vi "host.vi"() -> ()   [LabVIEW 2020]
uses:
  <vilib>/FPGAPlugInAG/cRIO-9035/niLvFpga_Open_cRIO-9035.vi
  <vilib>/rvi/interface/common/dynamic/niFpgaDynamicAddResources.vi
  <vilib>/rvi/interface/common/niFpgaWaitOnOcc.vi
  <vilib>/Utility/error.llb/Error Cluster From Error Code.vi
  <vilib>/rvi/errors/niLvFpgaAdjustHostInterfaceError.vi
  <vilib>/FPGAPlugInAG/Dynamic/niLvFpga_Run_Dynamic.vi
  <vilib>/FPGAPlugInAG/Dynamic/niLvFpga_Close_Dynamic.vi
  <vilib>/rvi/interface/nirviOpenFPGA/nirviOpenFPGA.xnode
  FPGA Bitfiles/fftfpgaapplicati_FPGATarget_FFT2_yc4HosK7ewc.lvbitx
  FFT.vi
  <vilib>/rvi/interface/nirviMethod/nirviMethod.xnode
  <vilib>/rvi/interface/nirviCloseFPGA/nirviCloseFPGA.xnode
  <vilib>/rvi/errors/niLvFpgaMergeErrorWithErrorCode.vi
  <vilib>/FPGAPlugInAG/Dynamic/niLvFpga_ReadFifo_Dynamic.vi
  <vilib>/Analysis/NI_AALPro.lvlib
  <vilib>/FPGAPlugInAG/Dynamic/niLvFpga_StartFifo_Dynamic.vi
  <vilib>/FPGAPlugInAG/Dynamic/niLvFpga_ConfigureFifo_Dynamic.vi
  <vilib>/FPGAPlugInAG/Dynamic/niLvFpga_WriteFifo_Dynamic.vi
panel:
  out "target to hostActual Depth 4":u32
  out "imag_Actual Depth 3":u32
  out "real actual depth":u32
  out "Actual Depth host to target":u32
  out "imaginary":fxp<+/-,32,21>[](array[numeric])
  out "real remain 1st":u32
  out "img remain 1st":u32
  out "data collrection remain 2nd":u32
  out "data collection remain 1st":u32
  out "FF T time remain 2nd":u32
  out "FFt time remain 1st":u32
  out "real remain 2nd":u32
  out "img remain 2nd":u32
  out "target to host remain 2nd":u32
  out "Empty Elements Remaining\nhost to target":u32
  out "signal_target_to_host_fixed size(s)":i32
  out "target to host remain 1st":u32
  out "Array":fxp<+/-,24,7>[](array[numeric])
  out "signal target to host":dbl[][](graph)
  out "data collection time":u32[](array[numeric])
  out "FFT time":u32[](array[numeric])
  out "signal_target_to_host_fixed":fxp<+/-,24,7>[](array[numeric])
  out "real array size":i32
  out "real Fixed":fxp<+/-,32,21>[](array[numeric])
  out "detrend acc":dbl[](graph)
  out "acc":dbl[](graph)
  out "samples":i32
  out "Waveform Graph":dbl[][](graph)
  out "input signal":T1(graph)
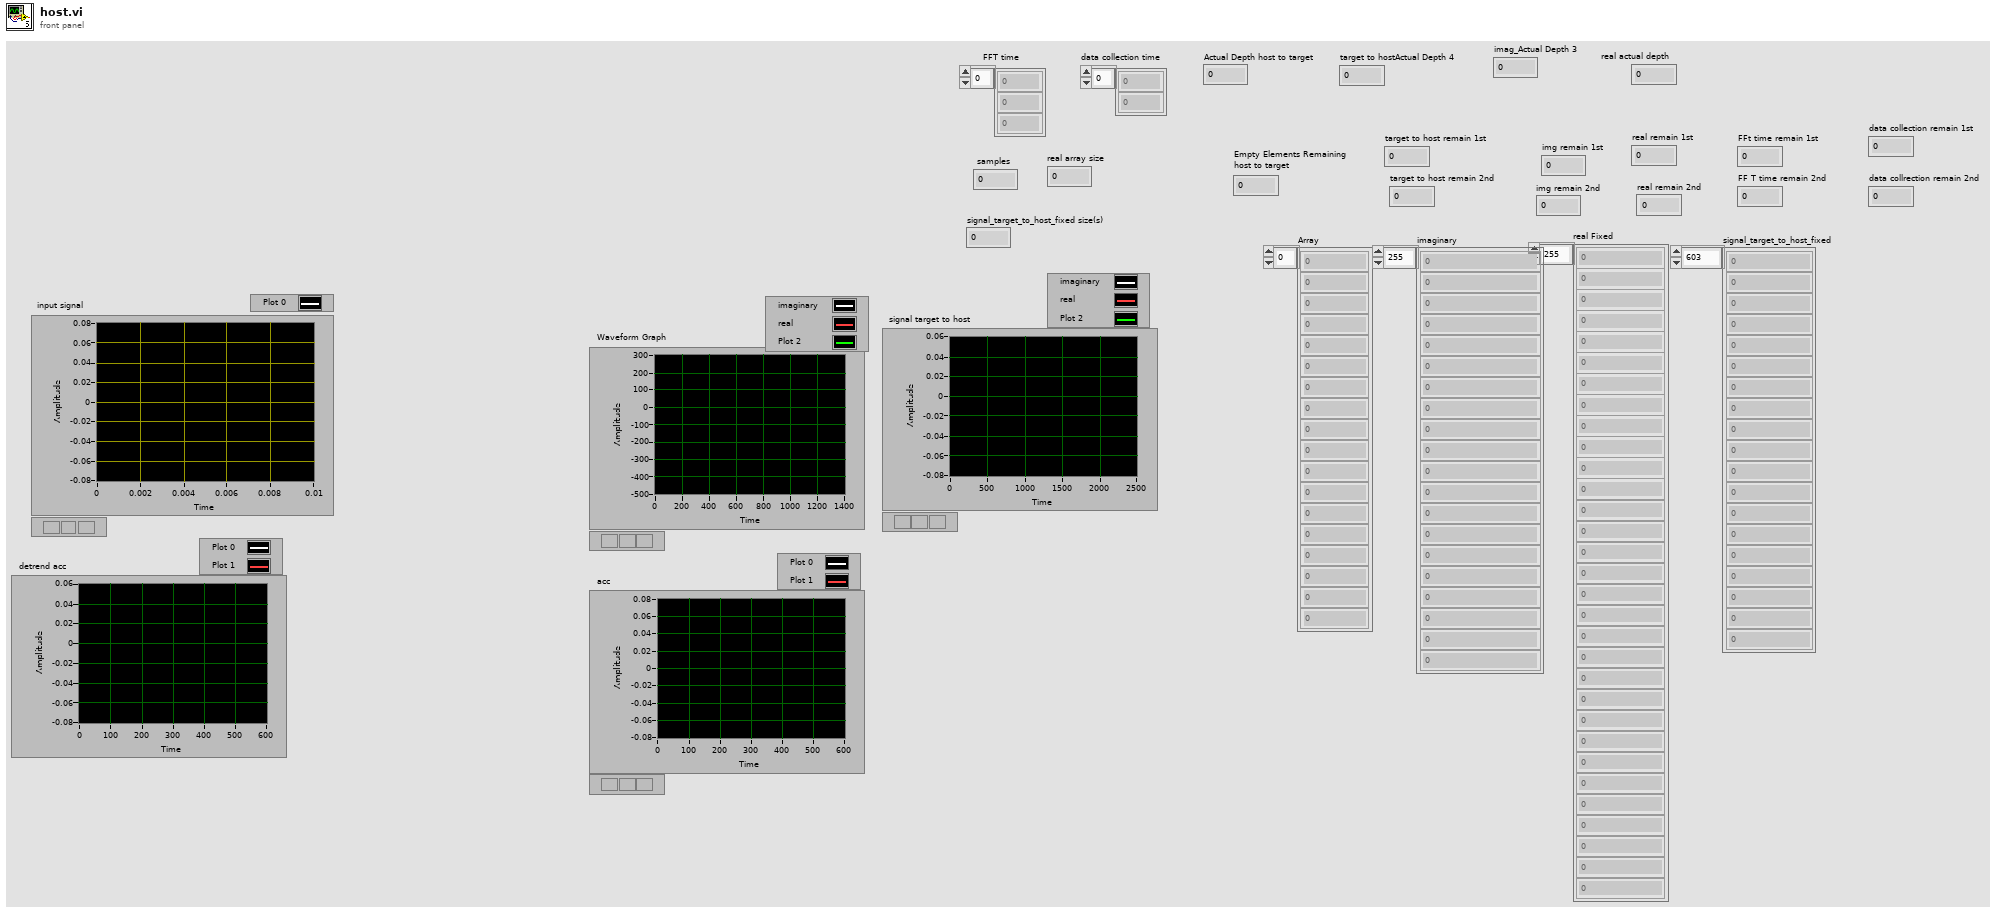
[diagram p1: front panel]
types:
  T1 = cluster{"array type (2D Dbl)":dbl[], "array type (2D Dbl)":dbl[]}
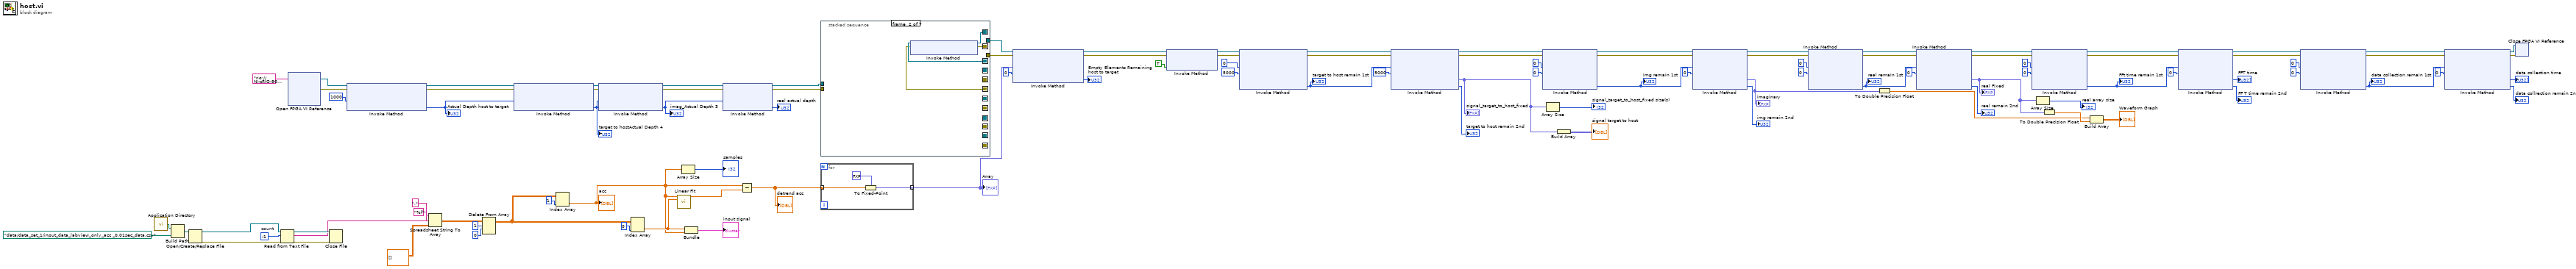
[diagram p0: block diagram]
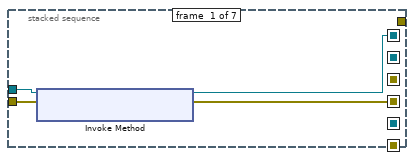
[diagram p2: hidden frame]
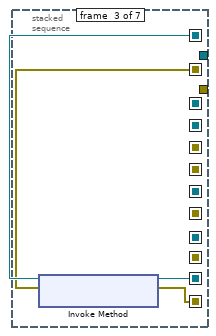
[diagram p3: hidden frame]
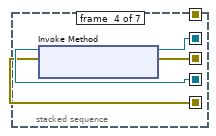
[diagram p4: hidden frame]
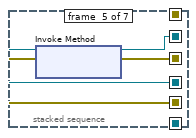
[diagram p5: hidden frame]
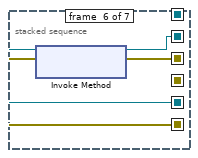
[diagram p6: hidden frame]
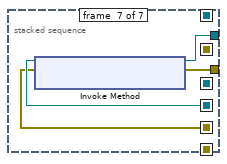
[diagram p7: hidden frame]
diagram:
  w97 = -1  # count
  n1 = call <vilib>:"Application Directory.vi"() -> ("Application Directory"=w101:path)
  n2 = Build Path(base path=w101, name or relative path=path "data/data_set_1/input_data_labview_only_acc _0.01sec_data.csv" ("default name")) -> (appended path=w100:path)
  n3 = Open/Create/Replace File(file path (use dialog)=w100) -> (refnum out=w105:refnum<file>, error out=w106:errorcluster)  [unwired: 5 in, 1 out]
  n4 = Read from Text File(file (use dialog)=w105, count=w97, error in=w106) -> (refnum out=w104:refnum<file>, text=w102:string, error out=w103:errorcluster)  [unwired: 1 in, 1 out]
  n5 = xnode "Open FPGA VI Reference"("resource name"=tag "rio://NI-cRIO-9035-01B68DD0/RIO0") -> ("FPGA VI Reference Out"=w10:refnum<k20>, "error out"=w9:errorcluster)  [unwired: 1 in]
  n6 = Close File(refnum=w104, error in=w103) -> ()  [unwired: 2 out]
  n7 = xnode "Invoke Method"("FPGA VI Reference In"=w10, "error in"=w9, "Requested Depth"=u32 1000) -> ("FPGA VI Reference Out"=w8:refnum<k20>, "error out"=w7:errorcluster, "Actual Depth"=w14:u32)
  "Actual Depth host to target" <- w14
  n8 = Spreadsheet String To Array(delimiter (Tab)=",", format string="%f", spreadsheet string=w102, array type (2D Dbl)=dbl[][] []) -> (array=w94:dbl[][])
  n9 = Delete From Array(array=w94, length=1, index (row)=0) -> (array with subset deleted=w89:dbl[][])  [unwired: 1 in, 1 out]
  n10 = xnode "Invoke Method"("FPGA VI Reference In"=w8, "error in"=w7, "Requested Depth"=w14) -> ("FPGA VI Reference Out"=w6:refnum<k20>, "error out"=w5:errorcluster, "Actual Depth"=w13:u32)
  "target to hostActual Depth 4" <- w13
  n11 = Index Array(array=w89, index (col)=1 ("disabled index (col)")) -> (element=w71:dbl[])  [unwired: 1 in]
  "acc" <- w71
  n12 = xnode "Invoke Method"("FPGA VI Reference In"=w6, "error in"=w5, "Requested Depth"=w13) -> ("FPGA VI Reference Out"=w4:refnum<k20>, "error out"=w3:errorcluster, "Actual Depth"=w12:u32)
  "imag_Actual Depth 3" <- w12
  n13 = Index Array(array=w89, index (col)=0 ("disabled index (col)")) -> (element=w74:dbl[])  [unwired: 1 in]
  n14 = call <vilib>:"Linear Fit.vi"("Y"=w71, "X"=w74) -> ("Best Linear Fit"=w72:dbl[])  [unwired: 9 in, 4 out]
  n15 = Array Size(array=w71) -> (size(s)=→"samples":i32)
  n16 = Bundle("array type (2D Dbl)"=w74, "array type (2D Dbl)"=w71) -> (→"input signal":T1)  [unwired: 1 in]
  n17 = xnode "Invoke Method"("FPGA VI Reference In"=w4, "error in"=w3, "Requested Depth"=w12) -> ("FPGA VI Reference Out"=w2:refnum<k20>, "error out"=w1:errorcluster, "Actual Depth"=→"real actual depth":u32)
  n18 = Subtract(x=w71, y=w72) -> (x-y=w73:dbl[])
  "detrend acc" <- w73
  n19 = stacked-sequence {
    seq-local: [w108 _ _ _ _ _ _] -> [_ w114 _ _ _ _ _]
    seq-local: [w107 _ _ _ _ _ _] -> [_ w113 _ _ _ _ _]
    seq-local: [_ w112 _ _ _ _ _] -> [_ _ w118 _ _ _ _]
    seq-local: [_ w111 _ _ _ _ _] -> [_ _ w117 _ _ _ _]
    seq-local: [_ _ w116 _ _ _ _] -> [_ _ _ w122 _ _ _]
    seq-local: [_ _ w115 _ _ _ _] -> [_ _ _ w121 _ _ _]
    seq-local: [_ _ _ w120 _ _ _] -> [_ _ _ _ w126 _ _]
    seq-local: [_ _ _ w119 _ _ _] -> [_ _ _ _ w125 _ _]
    seq-local: [_ _ _ _ w124 _ _] -> [_ _ _ _ _ w130 _]
    seq-local: [_ _ _ _ w123 _ _] -> [_ _ _ _ _ w129 _]
    seq-local: [_ _ _ _ _ w128 _] -> [_ _ _ _ _ _ w134]
    seq-local: [_ _ _ _ _ w127 _] -> [_ _ _ _ _ _ w133]
    tunnel: w2 -> [w110 _ _ _ _ _ _]
    tunnel: w1 -> [w109 _ _ _ _ _ _]
    tunnel: [_ _ _ _ _ _ w132] -> w34
    tunnel: [_ _ _ _ _ _ w131] -> w33
    frame #0 {
      n20 = xnode "Invoke Method"("FPGA VI Reference In"=w110, "error in"=w109) -> ("FPGA VI Reference Out"=w108:refnum<k20>, "error out"=w107:errorcluster)
    }
    frame #1 {
      n21 = xnode "Invoke Method"("FPGA VI Reference In"=w114, "error in"=w113) -> ("FPGA VI Reference Out"=w112:refnum<k20>, "error out"=w111:errorcluster)
    }
    frame #2 {
      n22 = xnode "Invoke Method"("FPGA VI Reference In"=w118, "error in"=w117) -> ("FPGA VI Reference Out"=w116:refnum<k20>, "error out"=w115:errorcluster)
    }
    frame #3 {
      n23 = xnode "Invoke Method"("FPGA VI Reference In"=w122, "error in"=w121) -> ("FPGA VI Reference Out"=w120:refnum<k20>, "error out"=w119:errorcluster)
    }
    frame #4 {
      n24 = xnode "Invoke Method"("FPGA VI Reference In"=w126, "error in"=w125) -> ("FPGA VI Reference Out"=w124:refnum<k20>, "error out"=w123:errorcluster)
    }
    frame #5 {
      n25 = xnode "Invoke Method"("FPGA VI Reference In"=w130, "error in"=w129) -> ("FPGA VI Reference Out"=w128:refnum<k20>, "error out"=w127:errorcluster)
    }
    frame #6 {
      n26 = xnode "Invoke Method"("FPGA VI Reference In"=w134, "error in"=w133) -> ("FPGA VI Reference Out"=w132:refnum<k20>, "error out"=w131:errorcluster)
    }
  }
  n27 = for {
    tunnel: [w136] -> w62 mode=indexing
    tunnel: w73 -> [w135] mode=indexing
    n28 = To Fixed-Point(fixed-point type=fxp<+/-,24,7> 0.0 ("f"), number=w135) -> (fixed-point=w136:fxp<+/-,24,7>)
  }
  "Array" <- w62
  n29 = xnode "Invoke Method"("FPGA VI Reference In"=w34, "error in"=w33, "Data"=w62, "Timeout (ms)"=0) -> ("FPGA VI Reference Out"=w86:refnum<k20>, "error out"=w85:errorcluster, "Empty Elements Remaining"=→"Empty Elements Remaining\nhost to target":u32)
  n30 = xnode "Invoke Method"("FPGA VI Reference In"=w86, "error in"=w85, "Wait Until Done (F)"=TRUE) -> ("FPGA VI Reference Out"=w63:refnum<k20>, "error out"=w64:errorcluster)
  n31 = xnode "Invoke Method"("FPGA VI Reference In"=w63, "error in"=w64, "Number of Elements"=u32 0, "Timeout (ms)"=5000) -> ("FPGA VI Reference Out"=w66:refnum<k20>, "error out"=w65:errorcluster, "Elements Remaining"=w31:u32)  [unwired: 1 out]
  "target to host remain 1st" <- w31
  n32 = xnode "Invoke Method"("FPGA VI Reference In"=w66, "error in"=w65, "Number of Elements"=w31, "Timeout (ms)"=5000) -> ("FPGA VI Reference Out"=w29:refnum<k20>, "error out"=w28:errorcluster, "Data"=w43:fxp<+/-,24,7>[], "Elements Remaining"=→"target to host remain 2nd":u32)
  "signal_target_to_host_fixed" <- w43
  n33 = xnode "Invoke Method"("FPGA VI Reference In"=w29, "error in"=w28, "Number of Elements"=u32 0, "Timeout (ms)"=0) -> ("FPGA VI Reference Out"=w25:refnum<k20>, "error out"=w24:errorcluster, "Elements Remaining"=w23:u32)  [unwired: 1 out]
  "img remain 1st" <- w23
  n34 = Array Size(array=w43) -> (size(s)=→"signal_target_to_host_fixed size(s)":i32)
  n35 = Build Array(w43) -> (→"signal target to host":fxp<+/-,24,7>[][])
  n36 = xnode "Invoke Method"("FPGA VI Reference In"=w25, "error in"=w24, "Number of Elements"=w23, "Timeout (ms)"=0) -> ("FPGA VI Reference Out"=w22:refnum<k20>, "error out"=w21:errorcluster, "Data"=w30:fxp<+/-,32,21>[], "Elements Remaining"=→"img remain 2nd":u32)
  "imaginary" <- w30
  n37 = xnode "Invoke Method"("FPGA VI Reference In"=w22, "error in"=w21, "Number of Elements"=u32 0, "Timeout (ms)"=0) -> ("FPGA VI Reference Out"=w20:refnum<k20>, "error out"=w19:errorcluster, "Elements Remaining"=w16:u32)  [unwired: 1 out]
  "real remain 1st" <- w16
  n38 = To Double Precision Float(number=w30) -> (double precision float=w67:dbl[])
  n39 = xnode "Invoke Method"("FPGA VI Reference In"=w20, "error in"=w19, "Number of Elements"=w16, "Timeout (ms)"=0) -> ("FPGA VI Reference Out"=w81:refnum<k20>, "error out"=w80:errorcluster, "Data"=w69:fxp<+/-,32,21>[], "Elements Remaining"=→"real remain 2nd":u32)
  "real Fixed" <- w69
  n40 = xnode "Invoke Method"("FPGA VI Reference In"=w81, "error in"=w80, "Number of Elements"=u32 0, "Timeout (ms)"=0) -> ("FPGA VI Reference Out"=w59:refnum<k20>, "error out"=w58:errorcluster, "Elements Remaining"=w57:u32)  [unwired: 1 out]
  "FFt time remain 1st" <- w57
  n41 = Array Size(array=w69) -> (size(s)=→"real array size":i32)
  n42 = To Double Precision Float(number=w69) -> (double precision float=w68:dbl[])
  n43 = Build Array(w67, w68) -> (→"Waveform Graph":dbl[][])
  n44 = xnode "Invoke Method"("FPGA VI Reference In"=w59, "error in"=w58, "Number of Elements"=w57, "Timeout (ms)"=0) -> ("FPGA VI Reference Out"=w55:refnum<k20>, "error out"=w54:errorcluster, "Data"=→"FFT time":u32[], "Elements Remaining"=→"FF T time remain 2nd":u32)
  n45 = xnode "Invoke Method"("FPGA VI Reference In"=w55, "error in"=w54, "Number of Elements"=u32 0, "Timeout (ms)"=0) -> ("FPGA VI Reference Out"=w53:refnum<k20>, "error out"=w52:errorcluster, "Elements Remaining"=w51:u32)  [unwired: 1 out]
  "data collection remain 1st" <- w51
  n46 = xnode "Invoke Method"("FPGA VI Reference In"=w53, "error in"=w52, "Number of Elements"=w51, "Timeout (ms)"=0) -> ("FPGA VI Reference Out"=w41:refnum<k20>, "error out"=w40:errorcluster, "Data"=→"data collection time":u32[], "Elements Remaining"=→"data collrection remain 2nd":u32)
  n47 = xnode "Close FPGA VI Reference"("FPGA VI Reference In"=w41, "error in"=w40) -> ()  [unwired: 1 out]
